vi "日期字符串格式至时间格式转换(子VI).vi"(10 "数值":dbl, 11 "data[0]":string) -> (3 "time stamp":timestamp format="%<%Y/%m/%d %H:%M:%S>T")   [LabVIEW 2016, in "数据传输系统-04.lvlib"]
uses:
  <vilib>/Utility/miscctls.llb/LVDateTimeRec.ctl
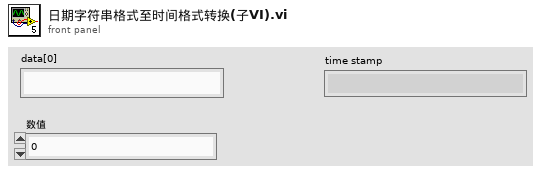
[diagram p1: front panel]
types:
  T1 = typedef "LVDateTimeRec.ctl" = cluster{"fractional second":dbl, "second":i32, "minute":i32, "hour":i32, "day of month":i32, "month":i32, "year":i32, "day of week":i32, "day of year":i32, "DST":i32}
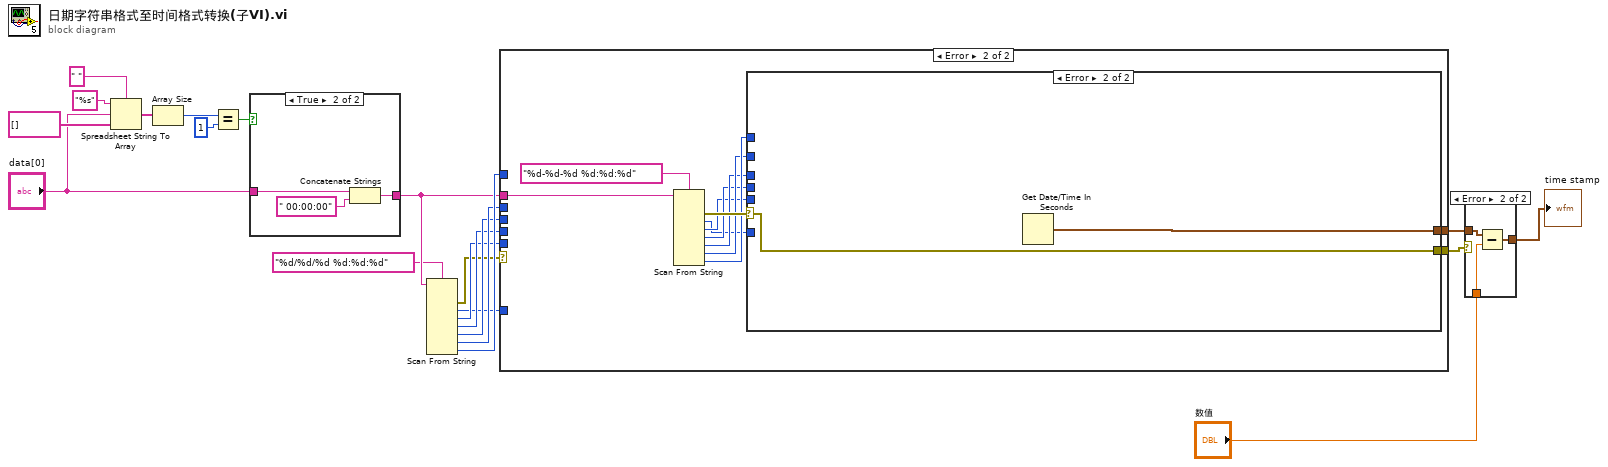
[diagram p0: block diagram]
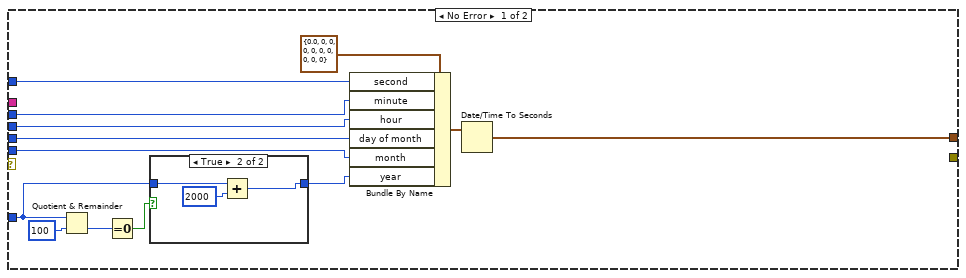
[diagram p4: hidden frame]
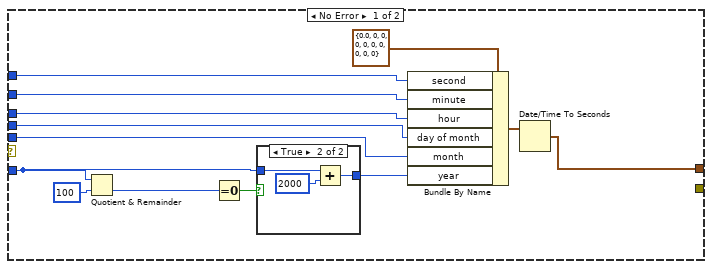
[diagram p6: hidden frame]
diagram:
  n1 = Spreadsheet String To Array(delimiter (Tab)=" " ("分隔符(Tab)"), format string="%s" ("格式字符串"), spreadsheet string="data[0]", array type (2D Dbl)=string[] []) -> (array=w11:string[])
  n2 = Array Size(array=w11) -> (size(s)=w10:i32)
  n3 = Equal?(x=w10, y=1) -> (x = y?=w8:bool)
  n4 = case shown="True" w8 {
    tunnel: "data[0]" -> [w22 w24]
    tunnel: [w22 w23] -> w6
    frame False {
    }
    frame True {
      n5 = Concatenate Strings(w24, " 00:00:00" ("字符串")) -> (w23:string)
    }
  }
  n6 = Scan From String(format string="%d/%d/%d %d:%d:%d" ("格式字符串"), input string=w6) -> (error out=w15:errorcluster, output 1=w16:i32, output 2=w17:i32, output 3=w18:i32, output 4=w19:i32, output 5=w20:i32, output 6=w21:i32)  [unwired: 8 in, 2 out]
  n7 = case shown="Error" w15 {
    tunnel: w21 -> [w37 _]
    tunnel: w20 -> [w36 _]
    tunnel: w19 -> [w35 _]
    tunnel: w18 -> [w34 _]
    tunnel: w17 -> [w33 _]
    tunnel: w16 -> [w29 _]
    tunnel: [w31 w50] -> w4
    tunnel: w6 -> [_ w53]
    tunnel: [_ w43] -> w1
    frame No Error {
      n8 = Quotient & Remainder(x=w29, y=100) -> (floor(x/y)=w28:i32)  [unwired: 1 out]
      n9 = Equal To 0?(x=w28) -> (x = 0?=w27:bool)
      n10 = case shown="True" w27 {
        tunnel: w29 -> [w39 w42]
        tunnel: [w39 w40] -> w26
        frame False {
        }
        frame True {
          n11 = Add(x=w42, y=2000) -> (x+y=w40:i32)
        }
      }
      n12 = Bundle By Name(cluster=T1 {"fractional second"=0.0, "second"=0, "minute"=0, "hour"=0, "day of month"=0, "month"=0, "year"=0, "day of week"=0, "day of year"=0, "DST"=0} ("日期时间记录"), "second"=w37, "minute"=w36, "hour"=w35, "day of month"=w34, "month"=w33, "year"=w26) -> (w38:T1)
      n13 = Date/Time To Seconds(2:w38) -> (0:w31:timestamp)  [unwired: 1 in]
    }
    frame Error {
      n14 = Scan From String(format string="%d-%d-%d %d:%d:%d" ("格式字符串"), input string=w53) -> (error out=w51:errorcluster, output 1=w44:i32, output 2=w45:i32, output 3=w46:i32, output 4=w47:i32, output 5=w48:i32, output 6=w49:i32)  [unwired: 8 in, 2 out]
      n15 = case shown="Error" w51 {
        selector: w51 -> [_ w71]
        tunnel: [w60 w72] -> w50
        tunnel: w49 -> [w59 _]
        tunnel: w48 -> [w58 _]
        tunnel: w47 -> [w57 _]
        tunnel: w46 -> [w56 _]
        tunnel: w45 -> [w55 _]
        tunnel: w44 -> [w54 _]
        tunnel: [_ w71] -> w43
        frame No Error {
          n16 = Quotient & Remainder(x=w54, y=100) -> (floor(x/y)=w63:i32)  [unwired: 1 out]
          n17 = Equal To 0?(x=w63) -> (x = 0?=w62:bool)
          n18 = case shown="True" w62 {
            tunnel: w54 -> [w67 w70]
            tunnel: [w67 w68] -> w61
            frame False {
            }
            frame True {
              n19 = Add(x=w70, y=2000) -> (x+y=w68:i32)
            }
          }
          n20 = Bundle By Name(cluster=T1 {"fractional second"=0.0, "second"=0, "minute"=0, "hour"=0, "day of month"=0, "month"=0, "year"=0, "day of week"=0, "day of year"=0, "DST"=0} ("日期时间记录"), "second"=w59, "minute"=w58, "hour"=w57, "day of month"=w56, "month"=w55, "year"=w61) -> (w66:T1)
          n21 = Date/Time To Seconds(2:w66) -> (0:w60:timestamp)  [unwired: 1 in]
        }
        frame Error {
          n22 = Get Date/Time In Seconds() -> (seconds since 1Jan1904=w72:timestamp)
        }
      }
    }
  }
  n23 = case shown="Error" w1 {
    tunnel: w4 -> [w73 w76]
    tunnel: [w73 w75] -> w3
    tunnel: "数值" -> [_ w74]
    frame No Error {
    }
    frame Error {
      n24 = Subtract(x=w76, y=w74) -> (x-y=w75:timestamp)
    }
  }
  "time stamp" <- w3
